vi "Draw Expanded Icons.vi"(4 "Expanded Types":T1[](array[typedef]), 6 "State":T7, 7 "Sizes":T6, 11 "Picture  In":picture) -> (3 "Picture":picture)   [LabVIEW 2020, in "FlexBlock.xnode"]
uses:
  FlexBlock.xnode
  State.ctl
  FlexBlocks/Type Descriptor.ctl
  FlexBlocks/Terminal Direction.ctl
  FlexBlocks/Value Mode.ctl
  FlexBlocks/Terminal State.ctl
  FlexBlocks/Special Terminal.ctl
  FlexBlocks/Errors.ctl
  <vilib>/picture/picture.llb/imagedata.ctl
  FlexBlocks/Calculated Sizes.ctl
  FlexBlocks/Size Constants.ctl
  FlexBlocks/FlexBlocks.lvlib
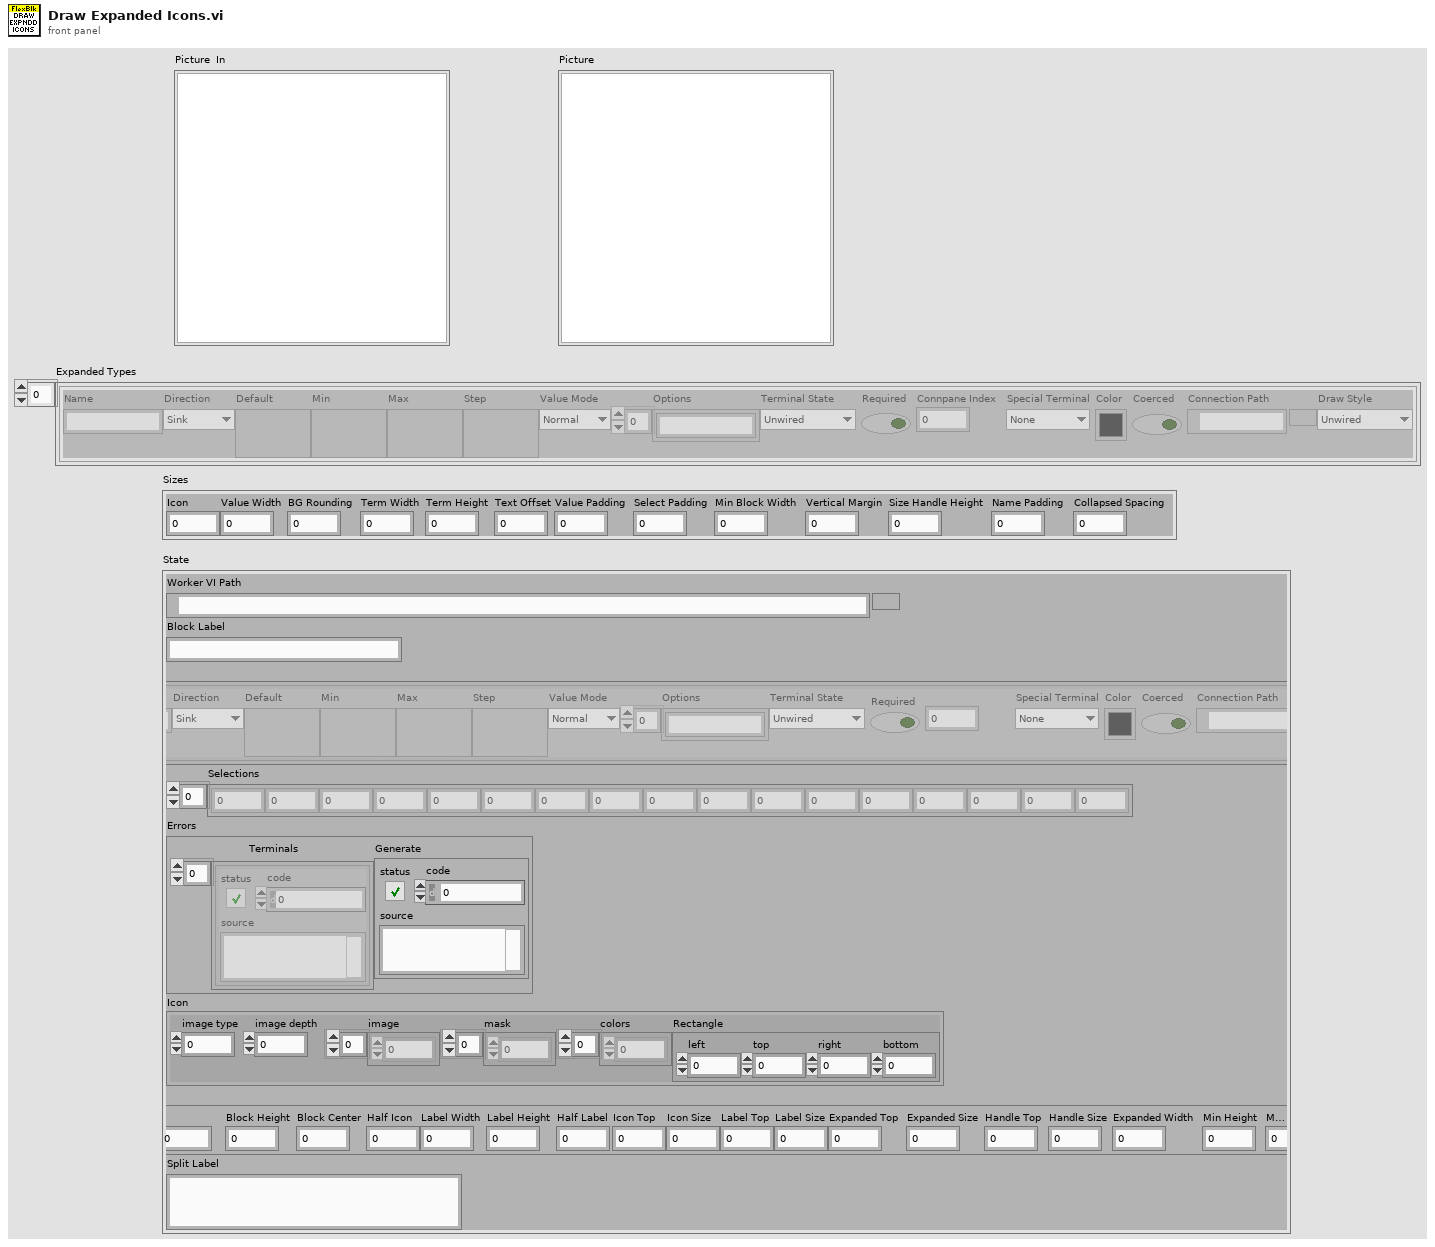
[diagram p1: front panel]
types:
  T1 = typedef "FlexBlocks.lvlib/Type Descriptor.ctl" = cluster{"Name":string, "Direction":T2, "Default":variant, "Min":variant, "Max":variant, "Step":variant, "Value Mode":T3, "Options":string[], "Terminal State":T4, "Required":bool, "Connpane Index":i32, "Special Terminal":T5, "Color":u32, "Coerced":bool, "Connection Path":path, "Draw Style":T4}
  T2 = typedef "FlexBlocks.lvlib/Terminal Direction.ctl" = enum16{"Sink", "Source"}
  T3 = typedef "FlexBlocks.lvlib/Value Mode.ctl" = enum16{"Normal", "Range", "Select"}
  T4 = typedef "FlexBlocks.lvlib/Terminal State.ctl" = enum16{"Unwired", "BadType", "BadRef", "Channel", "Value", "Control Ref"}
  T5 = typedef "FlexBlocks.lvlib/Special Terminal.ctl" = enum16{"None", "Action", "Init", "Tag", "State in", "State out", "Error"}
  T6 = typedef "FlexBlocks.lvlib/Size Constants.ctl" = cluster{"Icon":i32, "Value Width":i32, "BG Rounding":i32, "Term Width":i32, "Term Height":i32, "Text Offset":i32, "Value Padding":i32, "Select Padding":i32, "Min Block Width":i32, "Vertical Margin":i32, "Size Handle Height":i32, "Name Padding":i32, "Collapsed Spacing":i32}
  T7 = typedef "FlexBlock.xnode/State.ctl" = cluster{"Worker VI Path":path, "Block Label":string, "Types":T1[], "Selections":i32[], "Errors":T8, "Icon":T9, "Calcd Sizes":T10, "Split Label":string}
  T8 = typedef "FlexBlocks.lvlib/Errors.ctl" = cluster{"Terminals":errorcluster[], "Generate":errorcluster}
  T9 = typedef "imagedata.ctl" = cluster{"image type":i32, "image depth":i32, "image":u8[], "mask":u8[], "colors":u32[], "Rectangle":cluster{"left":i16, "top":i16, "right":i16, "bottom":i16}}
  T10 = typedef "FlexBlocks.lvlib/Calculated Sizes.ctl" = cluster{"Text Width":i32, "Text Height":i32, "Half Text":i32, "Block Width":i32, "Block Height":i32, "Block Center":i32, "Half Icon":i32, "Label Width":i32, "Label Height":i32, "Half Label":i32, "Icon Top":i32, "Icon Size":i32, "Label Top":i32, "Label Size":i32, "Expanded Top":i32, "Expanded Size":i32, "Handle Top":i32, "Handle Size":i32, "Expanded Width":i32, "Min Height":i32, "Max Height":i32}
  T11 = cluster{"left":i16, "top":i16, "right":i16, "bottom":i16}
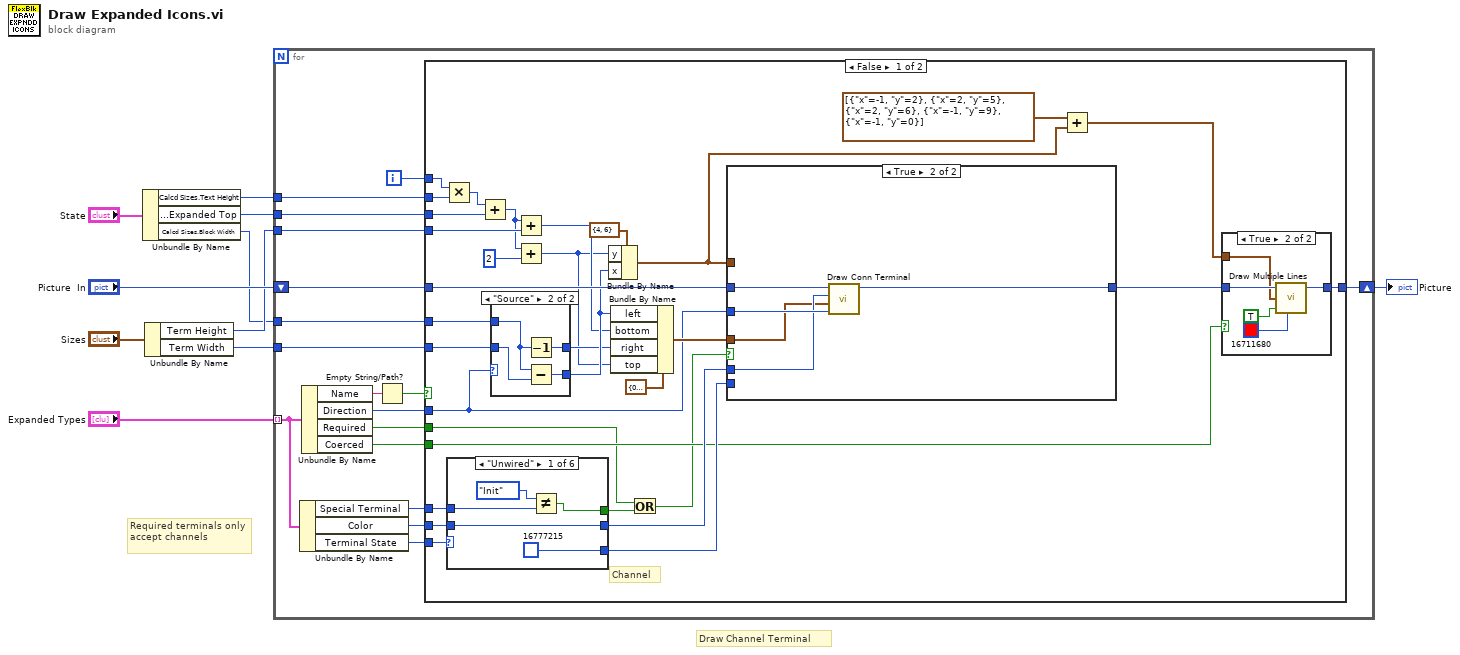
[diagram p0: block diagram]
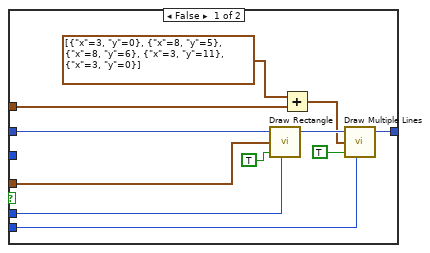
[diagram p2: hidden frame]
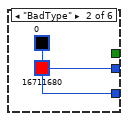
[diagram p4: hidden frame]
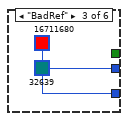
[diagram p5: hidden frame]
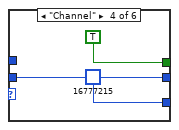
[diagram p6: hidden frame]
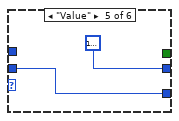
[diagram p7: hidden frame]
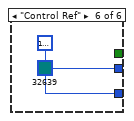
[diagram p8: hidden frame]
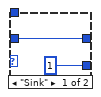
[diagram p9: hidden frame]
diagram:
  # "Draw Channel Terminal"
  # "Required terminals only accept channels"
  n1 = Unbundle By Name("State") -> ("Calcd Sizes.Text Height"=w2:i32, "Calcd Sizes.Expanded Top"=w1:i32, "Calcd Sizes.Block Width"=w3:i32)
  n2 = Unbundle By Name("Sizes") -> ("Term Height"=w4:i32, "Term Width"=w6:i32)
  n3 = for {
    shift-right: [w23] -> w9
    shift-left: "Picture  In" -> [w22]
    tunnel: "Expanded Types" -> [w26] mode=indexing
    tunnel: w6 -> [w19]
    tunnel: w4 -> [w17]
    tunnel: w3 -> [w16]
    tunnel: w2 -> [w15]
    tunnel: w1 -> [w14]
    i -> [w18]
    n4 = Unbundle By Name(w26) -> ("Special Terminal"=w11:T5, "Color"=w24:u32, "Terminal State"=w25:T4)
    n5 = Unbundle By Name(w26) -> ("Name"=w21:string, "Direction"=w27:T2, "Required"=w12:bool, "Coerced"=w13:bool)
    n6 = Empty String/Path?(string/path=w21) -> (empty?=w20:bool)
    n7 = case shown="False" w20 {
      tunnel: w27 -> [w31 _]
      tunnel: w25 -> [w59 _]
      tunnel: w24 -> [w58 _]
      tunnel: [w36 w104] -> w23
      tunnel: w22 -> [w56 w104]
      tunnel: w19 -> [w51 _]
      tunnel: w18 -> [w44 _]
      tunnel: w17 -> [w48 _]
      tunnel: w16 -> [w45 _]
      tunnel: w15 -> [w43 _]
      tunnel: w14 -> [w42 _]
      tunnel: w13 -> [w38 _]
      tunnel: w12 -> [w32 _]
      tunnel: w11 -> [w28 _]
      frame False {
        # "Channel"
        n8 = Multiply(x=w44, y=w43) -> (x*y=w41:i32)
        n9 = case shown="\"Unwired\"" w59 {
          tunnel: w58 -> [w86 _ _ w93 w94 _]
          tunnel: [w86 u32 0 ("color(black)") u32 16711680 ("color(black)") w93 u32 16777216 ("color(black)") u32 16777216 ("color(black)")] -> w55
          tunnel: [u32 16777215 ("color(black)") u32 16711680 ("color(black)") u32 32639 ("color(black)") u32 16777215 ("color(black)") w94 u32 32639 ("color(black)")] -> w54
          tunnel: [w82 _ _ TRUE _ _] -> w29
          tunnel: w28 -> [w84 _ _ _ _ _]
          frame "Unwired" {
            n10 = Not Equal?(x=Special_Terminal."Init", y=w84) -> (x != y?=w82:bool)
          }
          frame "BadType" {
          }
          frame "BadRef" {
          }
          frame "Channel" {
          }
          frame "Value" {
          }
          frame "Control Ref" {
          }
        }
        n11 = Add(x=w41, y=w42) -> (x+y=w40:i32)
        n12 = case shown="\"Source\"" w31 {
          tunnel: [i16 1 ("x") w102] -> w50
          tunnel: w51 -> [w98 w100]
          tunnel: [w98 w103] -> w49
          tunnel: w45 -> [_ w101]
          frame "Sink" {
          }
          frame "Source" {
            n13 = Decrement(x=w101) -> (x-1=w103:i32)
            n14 = Subtract(x=w101, y=w100) -> (x-y=w102:i32)
          }
        }
        n15 = Add(x=w40, y=w48) -> (x+y=w46:i32)
        n16 = Add(x=w40, y=2) -> (x+y=w39:i32)
        n17 = Bundle By Name(cluster=cluster{"x":i16, "y":i16} {"x"=4, "y"=6}, "y"=w39, "x"=w50) -> (w33:cluster{"x":i16, "y":i16})
        n18 = Bundle By Name(cluster=T11 {"left"=0, "top"=0, "right"=0, "bottom"=0} ("rect"), "left"=w50, "bottom"=w46, "right"=w49, "top"=w39) -> (w52:T11)
        n19 = Or(x=w32, y=w29) -> (x .or. y?=w30:bool)
        n20 = case shown="True" w30 {
          tunnel: w56 -> [w65 w75]
          tunnel: w55 -> [w64 w72]
          tunnel: w54 -> [w63 _]
          tunnel: w52 -> [w62 w71]
          tunnel: [w61 w74] -> w37
          tunnel: w33 -> [w60 _]
          tunnel: w31 -> [_ w73]
          frame False {
            n21 = call <vilib>:"Draw Rectangle.vi"("picture"=w65, "rect"=w62, "fill?(F)"=TRUE, "color(black)"=w64) -> ("new picture"=w69:picture)  [unwired: 5 in]
            n22 = Add(x=cluster{"x":i16, "y":i16}[] [{"x"=3, "y"=0}, {"x"=8, "y"=5}, {"x"=8, "y"=6}, {"x"=3, "y"=11}, {"x"=3, "y"=0}] ("line endpoints"), y=w60) -> (x+y=w67:cluster{"x":i16, "y":i16}[])
            n23 = call <vilib>:"Draw Multiple Lines.vi"("picture"=w69, "line endpoints"=w67, "fill?(F)"=TRUE, "color(black)"=w63) -> ("new picture"=w61:picture)  [unwired: 5 in]
          }
          frame True {
            n24 = call "Draw Conn Terminal.vi"("Direction"=w73, "Rect"=w71, "Type Color"=w72, "Picture  In"=w75) -> ("Picture"=w74:picture)  [unwired: 7 in]
          }
        }
        n25 = Add(x=cluster{"x":i16, "y":i16}[] [{"x"=-1, "y"=2}, {"x"=2, "y"=5}, {"x"=2, "y"=6}, {"x"=-1, "y"=9}, {"x"=-1, "y"=0}] ("line endpoints"), y=w33) -> (x+y=w34:cluster{"x":i16, "y":i16}[])
        n26 = case shown="True" w38 {
          tunnel: w37 -> [w76 w81]
          tunnel: [w76 w78] -> w36
          tunnel: w34 -> [_ w77]
          frame False {
          }
          frame True {
            n27 = call <vilib>:"Draw Multiple Lines.vi"("picture"=w81, "line endpoints"=w77, "fill?(F)"=TRUE, "color(black)"=u32 16711680) -> ("new picture"=w78:picture)  [unwired: 5 in]
          }
        }
      }
      frame True {
      }
    }
  }
  "Picture" <- w9
